vi "Format Message String.vi"(0 "Source":string="Fehler 333 tratt an der Fehlerquelle auf" caption="Quelle", 2 "Details":string="Ursache des Problem\nasdfasdf\tasdfaa sdfja ;sldjf;alskdjf;a lksjdf da ist viel mehr als das Auge im ersten Moment erfassen kann ;laiwje;fliajsd;flk ajsdlkfja psoieur a;lwdjf; alksjdf;alksdjf; alksedrfap oiwejf;alkw\nwerasdf\t3425 a b c d e f g h i j k l m n o p q\nafsdfasdfasdfasdfas asdf asdf\tasdfasd", 3 "String to Format (not a refnum)":refnum<vi> caption="String nach Format (kein Refnum)") -> (1 "message":string="OK" caption="Meldung", 5 "Bold Start":i32[](array[numeric]) caption="Fett Start", 6 "Bold Length":i32[](array[numeric]) caption="Fett Länge", 7 "Source Out":string="Fehler 333 tratt an der Fehlerquelle auf" caption="Quelle (Ausgang)", 8 "Details Out":string caption="Details Ausgang")   [LabVIEW 2009]
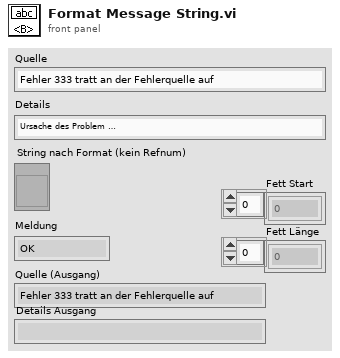
[diagram p1: front panel]
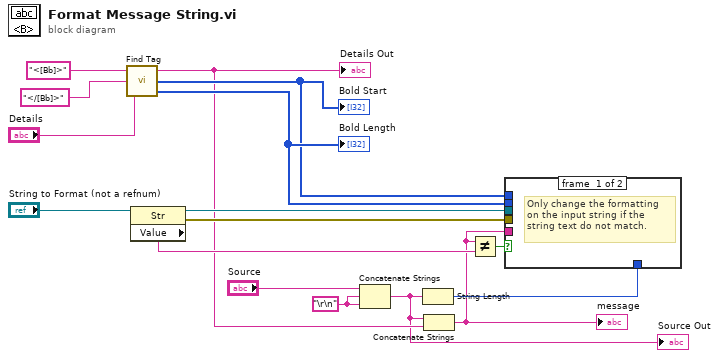
[diagram p0: block diagram]
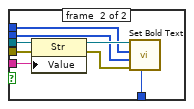
[diagram p2: hidden frame]
diagram:
  w14 = "\r\n"
  n1 = call "Find Tag.vi"("string"="Details", "close tag"="</[Bb]>" ("don't translate!"), "open tag"="<[Bb]>" ("don't translate!")) -> ("Length"=w13:i32[], "Start"=w12:i32[], "string out"=w6:string)
  "Bold Start" <- w12
  "Bold Length" <- w13
  "Details Out" <- w6
  n2 = property class="Str"(reference="String to Format (not a refnum)") -> (reference out=w10:refnum<vi>, error out=w9:errorcluster, "Value"=w8:string)  [unwired: 1 in]
  n3 = Concatenate Strings("Source", w14, w14) -> (w3:string)
  "Source Out" <- w3
  n4 = String Length(string=w3) -> (length=w5:i32)
  n5 = Concatenate Strings(w3, w6) -> (w4:string)
  "message" <- w4
  n6 = Not Equal?(x=w4, y=w8) -> (x != y?=w7:bool)
  n7 = case shown="True" w7 {
    tunnel: w13 -> [_ w22]
    tunnel: w12 -> [_ w21]
    tunnel: w10 -> [_ w20]
    tunnel: w9 -> [_ w19]
    tunnel: w4 -> [_ w18]
    tunnel: w5 -> [_ w17]
    frame #0 {
      # "Only change the formatting\non the input string if the \nstring text do not match."
    }
    frame #1 {
      n8 = property class="Str"(reference=w20, error in=w19, "Value"=w18) -> (reference out=w24:refnum<vi>, error out=w23:errorcluster)
      n9 = call "Set Bold Text.vi"("prefix adjustment"=w17, "error in"=w23, "Length"=w22, "Start"=w21, "text"=w24) -> ()  [unwired: 1 in, 1 out]
    }
  }
